vi "Divide.vi"(10 "d":i32, 11 "c":i32) -> (3 "function return":dbl)   [LabVIEW 2015, in "SimpleDLLSecond.lvlib"]
doc: "__declspec(dllexport) double Divide(double c, double d);"
uses:
  SimpleDLLSecond.lvlib
  SimpleDLLSecond.dll
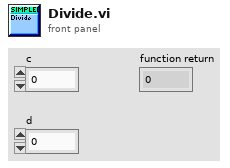
[diagram p1: front panel]
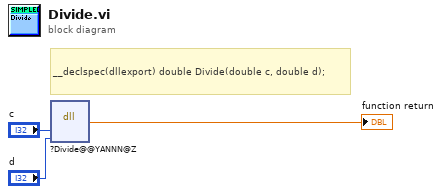
[diagram p0: block diagram]
diagram:
  # "__declspec(dllexport) double Divide(double c, double d);"
  n1 = dll-call lib="C:/Users/adahal/Desktop/AJ/LABVIEW/FirstDLL/SimpleDLLSecond.*" fn="?Divide@@YANNN@Z"("c"="c", "d"="d") -> (→"function return":dbl)  [unwired: 5 in, 2 out]
